vi "Format Number to Hz or kHz.vi"(8 "error in (no error)":errorcluster, 11 "Value":dbl) -> (0 "error out":errorcluster, 1 "Units":string, 2 "Value Out":string, 3 "Value Out (DBL)":dbl)   [LabVIEW 2018]
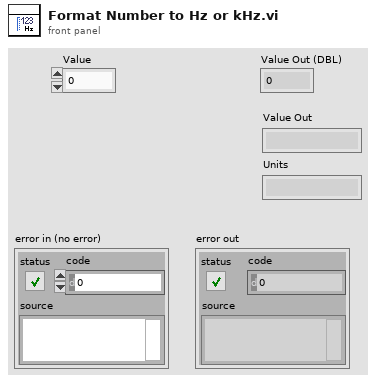
[diagram p1: front panel]
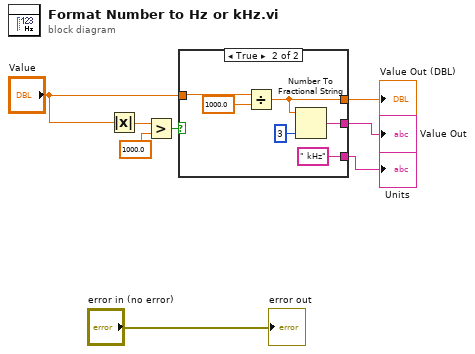
[diagram p0: block diagram]
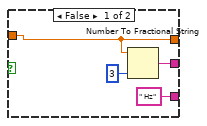
[diagram p2: hidden frame]
diagram:
  n1 = Absolute Value(x="Value") -> (abs(x)=w8:dbl)
  n2 = Greater?(x=w8, y=1000.0) -> (0:w6:bool)
  n3 = case shown="True" w6 {
    tunnel: "Value" -> [w10 w18]
    tunnel: [w10 w16] -> w4
    tunnel: [w11 w14] -> w3
    tunnel: [" Hz" " kHz"] -> w2
    frame False {
      n4 = Number To Fractional String(number=w10, precision (6)=i16 3) -> (F-format string=w11:string)  [unwired: 2 in]
    }
    frame True {
      n5 = Divide(x=w18, y=1000.0) -> (x/y=w16:dbl)
      n6 = Number To Fractional String(number=w16, precision (6)=i16 3) -> (F-format string=w14:string)  [unwired: 2 in]
    }
  }
  "Value Out" <- w3
  "Value Out (DBL)" <- w4
  "Units" <- w2
  "error out" <- "error in (no error)"
